vi "createEvents.vi"(8 "error in (no error)":errorcluster, 11 "MonoCommunicator in":refnum<class "MonoCommunicator.lvclass">) -> (0 "error out":errorcluster, 3 "MonoCommunicator out":refnum<class "MonoCommunicator.lvclass">)   [LabVIEW 2016, in "MonoCommunicator.lvclass"]
uses:
  MonoCommunicator.lvclass
  MonoCommunicator.lvclass/MonoCommunicator.ctl
  MonoPubSubData/MonoPubSubData.lvclass
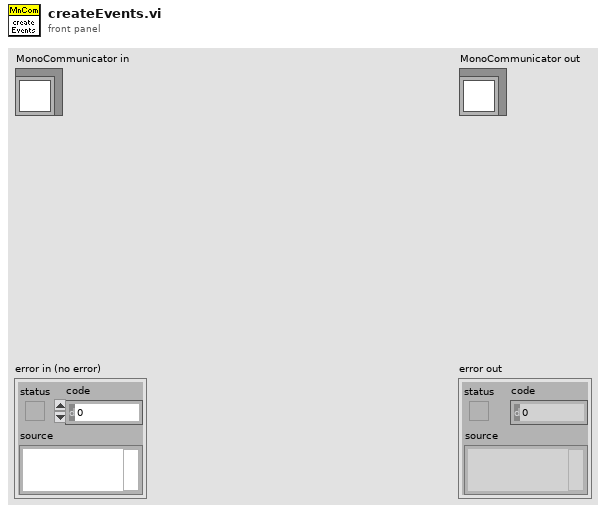
[diagram p1: front panel]
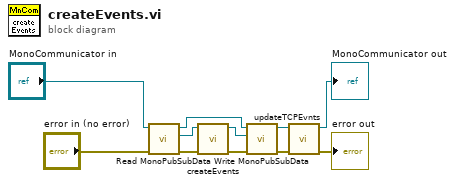
[diagram p0: block diagram]
diagram:
  n1 = call "Read MonoPubSubData.vi"("error in (no error)"="error in (no error)", "MonoCommunicator in"="MonoCommunicator in") -> ("error out"=w9:errorcluster, "MonoPubSubData.lvclass"=w8:refnum<class "MonoPubSubData.lvclass">, "MonoCommunicator out"=w6:refnum<class "MonoCommunicator.lvclass">)  [unwired: 7 in]
  n2 = call "createEvents.vi"("error in (no error)"=w9, "MonoPubSubData in"=w8) -> ("error out"=w7:errorcluster, "MonoPubSubData out"=w5:refnum<class "MonoPubSubData.lvclass">)  [unwired: 8 in]
  n3 = call "Write MonoPubSubData.vi"("error in (no error)"=w7, "MonoPubSubData.lvclass"=w5, "MonoCommunicator in"=w6) -> ("error out"=w4:errorcluster, "MonoCommunicator out"=w1:refnum<class "MonoCommunicator.lvclass">)  [unwired: 7 in]
  n4 = call "updateTCPEvnts.vi"("error in (no error)"=w4, "MonoCommunicator in"=w1) -> ("error out"=→"error out":errorcluster, "MonoCommunicator out"=→"MonoCommunicator out":refnum<class "MonoCommunicator.lvclass">)  [unwired: 8 in]
